vi "Destroy.vi"(8 "Error In":errorcluster, 11 "Session":refnum<class "Session.lvclass">) -> (0 "Error Out":errorcluster, 3 "labssh2 Shared Library":path)   [LabVIEW 2017, in "Toolkit.lvlib" / "Session.lvclass"]
uses:
  Session.lvclass
  Session.lvclass/Session.ctl
  Toolkit.lvlib
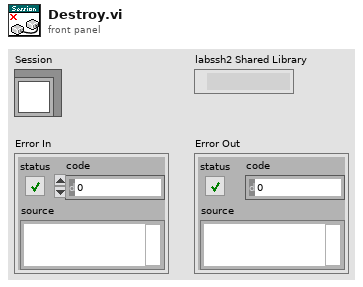
[diagram p1: front panel]
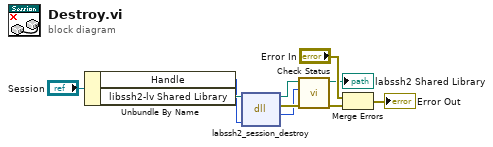
[diagram p0: block diagram]
diagram:
  n1 = Unbundle By Name("Session") -> ("Handle"=w7:u64, "libssh2-lv Shared Library"=w8:path)
  n2 = dll-call lib="D:/Users/cfield/Code/Field R&D Services/SSH/LabSSH2/LabVIEW/trunk/src/LabSSH2/Private/labssh2.*" fn="labssh2_session_destroy"(path in=w8, "handle"=w7) -> (path out=w4:path, error out=w5:errorcluster, "status"=w1:i32)  [unwired: 3 in]
  n3 = call "Check Status.vi"("Error In"=w5, "Status"=w1, "labssh2 Shared Library In"=w4) -> ("Error Out"=w2:errorcluster, "labssh2 Shared Library Out"=→"labssh2 Shared Library":path)  [unwired: 7 in]
  n4 = Merge Errors("Error In", w2) -> (→"Error Out":errorcluster)
